vi "AR Drone + Simple nav.vi"() -> ()   [LabVIEW 2014]
doc: "Very simple example showing how to use the base VIs to control the AR Drone and receive and display video data."
uses:
  Others/Control cluster.ctl
  <vilib>/LVH/AR Drone Toolkit/Decode NavData/Typedefs/NavData Demo.ctl
  Global.vi
  <vilib>/LVH/AR Drone Toolkit/AR Drone.lvlib
panel:
  in  "device ID":i32=3
  in  "milliseconds to wait":u32=5
  out "Delay (ms)":u32
  in  "Takeoff/Land":bool
  out "Video Stream 2":picture
  in  "Setup Parameters":T1={"Drone IP address"="192.168.1.1", "Home IP address"="192.168.1.2", "Flight Mode"=enum."INDOOR MODE", "Mounted Hull"=enum."INDOOR HULL", "Video Camera"=0, "Max Altitude (m)"=3.0, "Max Pitch and Roll Angle (deg)"=10.0, "Max Vertical Speed (m/s)"=0.7, "Max Yaw Speed (deg/s)"=100.0} {"Video Camera" items=["Bottom Camera"=1, "Front Camera"=0, "Front in Bottom"=3, "Bottom in Front"=2]}
  in  "stop":bool
  out "Loop error":errorcluster
  out "Loop count":i32
  out "Battery Remaining 2":dbl(slide) scale=0.0..100.0
  out "NavData Out 2":T2
  out "Control Cluster":T3 {"Yaw Speed" scale=-1.0..1.0; "Vertical Speed" scale=-1.0..1.0; "Pitch" scale=-1.0..1.0; "Roll" scale=-1.0..1.0}
  in  "Emergency Landing":bool
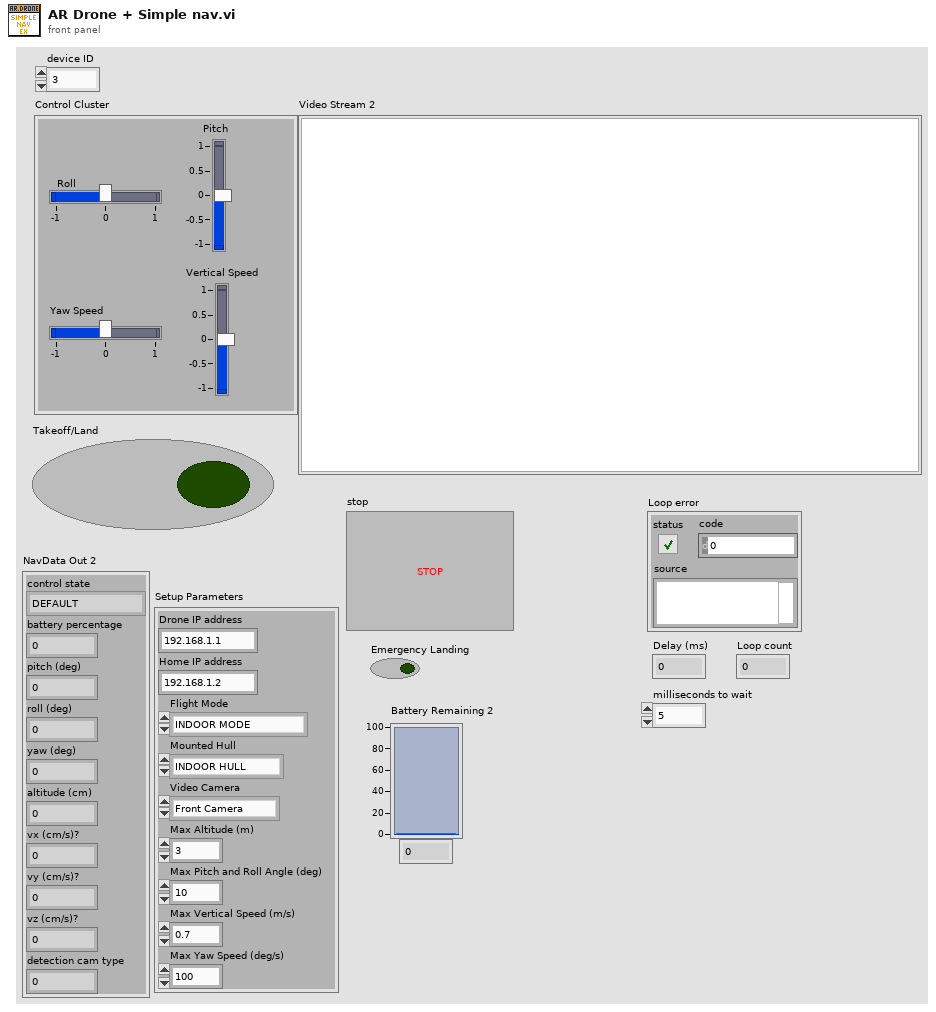
[diagram p1: front panel]
types:
  T1 = cluster{"Drone IP address":string, "Home IP address":string, "Flight Mode":enum8{"OUTDOOR MODE", "INDOOR MODE"}, "Mounted Hull":enum8{"OUTDOOR HULL", "INDOOR HULL"}, "Video Camera":u8, "Max Altitude (m)":sgl, "Max Pitch and Roll Angle (deg)":sgl, "Max Vertical Speed (m/s)":sgl, "Max Yaw Speed (deg/s)":sgl}
  T2 = typedef "AR Drone.lvlib/NavData Demo.ctl" = cluster{"control state":enum32{"DEFAULT", "INIT", "LANDING", "FLYING", "HOVERING", "TEST", "TRANS_TAKEOFF", "TRANS_GOTOFIX", "TRANS_LANDING"}, "battery percentage":u32, "pitch (deg)":sgl, "roll (deg)":sgl, "yaw (deg)":sgl, "altitude (cm)":u32, "vx (cm/s)?":sgl, "vy (cm/s)?":sgl, "vz (cm/s)?":sgl, "detection cam type":u32}
  T3 = typedef "Control cluster.ctl" = cluster{"Roll":sgl, "Pitch":sgl, "Vertical Speed":sgl, "Yaw Speed":sgl}
  T4 = typedef "AR Drone.lvlib/AR Drone Resource.ctl" = cluster{"UDP Control Connection":refnum<k16>, "UDP NavData Connection":refnum<k16>, "UDP Video Connection (Drone 1.0)":refnum<k16>, "TCP Video Connection (Drone 2.0)":refnum<k5>, "TCP Control Port Connection":refnum<k5>, "Drone IP address":string, "Drone Command Port":u16, "Drone NavData Port":u16, "Drone Vid Stream Port":u16, "Drone TCP Control Port":u16, "Home IP address":string, "Home Command Port":u16, "Home NavData Port":u16, "Home Vid Stream Port":u16, "Drone Version":i32, "Drone Index":i32, "Command Sequence":i32}
  T5 = cluster{"button 1":bool, "button 2":bool, "button 3":bool, "button 4":bool}
  T6 = cluster{"Roll":dbl, "Pitch":dbl, "Vertical Speed":dbl, "Yaw Speed":dbl}
  T7 = cluster{"Roll":sgl, "Pitch":sgl, "Vertical Speed":sgl, "Yaw Speed":sgl}
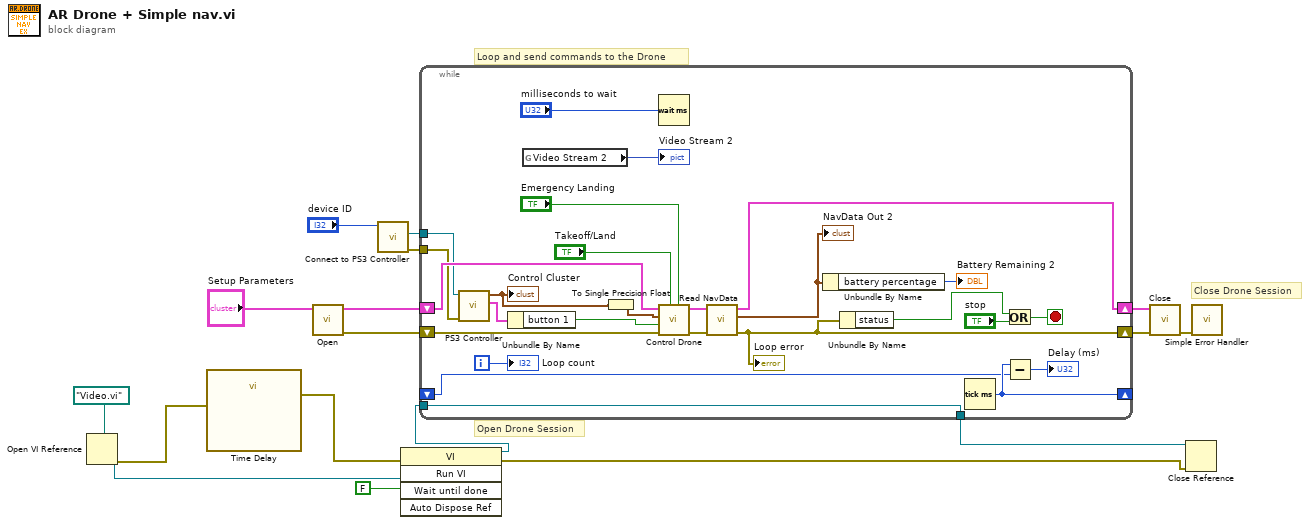
[diagram p0: block diagram]
diagram:
  # "Close Drone Session"
  # "Loop and send commands to the Drone"
  # "Open Drone Session"
  n1 = Open VI Reference(vi path=path "Video.vi") -> (vi reference=w8:refnum<vi>, error out=w2:errorcluster)  [unwired: 5 in]
  n2 = call "Time Delay"("error in (no error)"=w2) -> ("error out"=w1:errorcluster)  [unwired: 10 in]
  n3 = call <vilib>:"Open.vi"("Setup Parameters"="Setup Parameters") -> ("error out"=w15:errorcluster, "AR Drone Resource"=w11:T4)  [unwired: 9 in]
  n4 = call "Connect to PS3 Controller.vi"("device ID"="device ID") -> ("error out"=w12:errorcluster, "device ID 2"=w14:refnum<k1>)  [unwired: 7 in, 1 out]
  n5 = invoke class="VI" method="Run VI"(reference=w8, error in=w1, "Wait until done"=FALSE) -> (reference out=w7:refnum<vi>, error out=w5:errorcluster)  [unwired: 2 in, 3 out]
  n6 = while {
    shift-right: [w43] -> w17
    shift-left: w11 -> [w41]
    shift-right: [w36] -> w10
    shift-left: w15 -> [w42]
    tunnel: w14 -> [w39]
    tunnel: w12 -> [w38]
    shift-right: [w23] -> _
    shift-left: _ -> [w22]
    tunnel: w7 -> [w20]
    tunnel: [w20] -> w6
    i -> [w40]
    stop <- w37 stop-if-true
    n7 = call "PS3 Controller.vi"("error in (no error)"=w38, "device ID"=w39) -> ("Buttons control"=w34:T5, "Control cluster"=w19:T6)  [unwired: 6 in, 2 out]
    "Control Cluster" <- w19
    n8 = Unbundle By Name(w34) -> ("button 1"=w33:bool)
    n9 = global read "Global.vi" "Video Stream 2"() -> (→"Video Stream 2":picture)
    n10 = To Single Precision Float(number=w19) -> (single precision float=w18:T7)
    n11 = Wait (ms)(milliseconds to wait="milliseconds to wait") -> ()  [unwired: 1 out]
    n12 = call <vilib>:"Control Drone.vi"("Emergency Landing"="Emergency Landing", "Takeoff/Land"="Takeoff/Land", "error in (no error)"=w42, "Hover"=w33, "Control Cluster"=w18, "AR Drone Resource"=w41) -> ("error out"=w31:errorcluster, "AR Drone Resource Out"=w32:T4)  [unwired: 4 in]
    n13 = call <vilib>:"Read NavData.vi"("error in (no error)"=w31, "AR Drone Resource"=w32) -> ("error out"=w36:errorcluster, "NavData Out"=w24:T2, "AR Drone Resource Out"=w43:T4)  [unwired: 7 in]
    "Loop error" <- w36
    "NavData Out 2" <- w24
    n14 = Unbundle By Name(w24) -> ("battery percentage"=→"Battery Remaining 2":u32)
    n15 = Unbundle By Name(w36) -> ("status"=w27:bool)
    n16 = Tick Count (ms)() -> (millisecond timer value=w23:u32)
    n17 = Or(x=w27, y="stop") -> (x .or. y?=w37:bool)
    n18 = Subtract(x=w23, y=w22) -> (x-y=→"Delay (ms)":u32)
    "Loop count" <- w40
  }
  n19 = call <vilib>:"Close.vi"("error in (no error)"=w10, "AR Drone Resource"=w17) -> ("error out"=w16:errorcluster)  [unwired: 9 in]
  n20 = Close Reference(reference=w6, error in (no error)=w5) -> ()  [unwired: 1 out]
  n21 = call <vilib>:"Simple Error Handler.vi"("error in (no error)"=w16) -> ()  [unwired: 4 in, 5 out]
